vi "User Event Tester.vi"(8 "error in (no error)":errorcluster) -> (0 "error out":errorcluster)   [LabVIEW 2020]
uses:
  Support/Stop User Event/Controls/User event Actions.ctl
  Support/Stop User Event/User Event - Stop.lvlib
  Support/Modules Template/Module Template.lvlib
panel:
  in  "OK Button":bool
  in  "STOP":bool
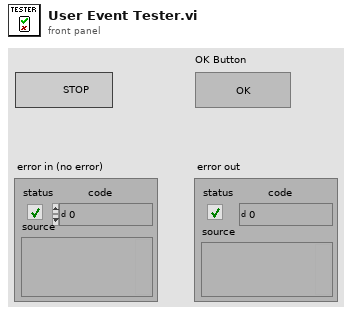
[diagram p1: front panel]
types:
  T1 = typedef "User Event - Stop.lvlib/User event Actions.ctl" = enum16{"Create", "Get Reference", "Fire Stop Event", "Destroy"}
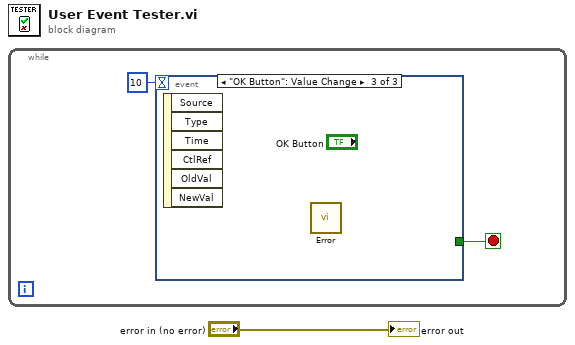
[diagram p0: block diagram]
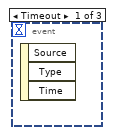
[diagram p2: hidden frame]
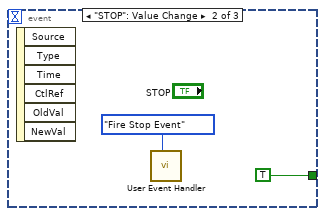
[diagram p3: hidden frame]
diagram:
  n1 = while {
    stop <- w2 stop-if-true
    n2 = event shown="[2] \"OK Button\": Value Change" {
      selector: _ -> [_ _ _]
      dyn-events: _ -> [_ _ _]
      timeout: 10 -> [_ _ _]
      tunnel: [_ TRUE _] -> w2
      event Timeout {
        n3 = event-data() -> ()  [unwired: 1 in, 3 out]
      }
      event "STOP": Value Change {
        n4 = event-data() -> ()  [unwired: 1 in, 6 out]
        n5 = call "User Event Handler.vi"("User Event Action"=User_event_Actions."Fire Stop Event") -> ()  [unwired: 9 in, 2 out]
      }
      event "OK Button": Value Change {
        n6 = event-data() -> ()  [unwired: 1 in, 6 out]
        n7 = call "Error.vi"() -> ()  [unwired: 11 in, 1 out]
      }
    }
  }
  "error out" <- "error in (no error)"
